vi "SetupDigitalPattern.vi"(6 "PatternfileName":string="Pattern.digipat", 8 "error in (no error)":errorcluster, 9 "DigitalWaveformName":string, 10 "pin list":string, 11 "IVI Refnum in":refnum<k15>) -> (0 "error out":errorcluster, 3 "IVI Refnum out":refnum<k15>)   [LabVIEW 2023]
uses:
  <instrlib>/niDigital/niDigital.llb/niDigital Load Specifications Levels and Timing (Single).vi
  <instrlib>/niDigital/niDigital.llb/niDigital Create Capture Waveform (Parallel).vi
  <instrlib>/niDigital/niDigital.llb/niDigital Create Source Waveform (Parallel).vi
  <instrlib>/niDigital/niDigital.llb/niDigital Write Source Waveform (Broadcast U32).vi
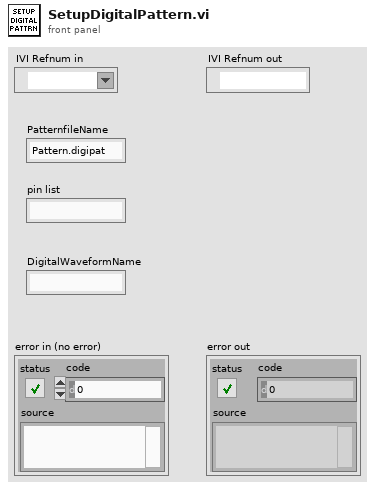
[diagram p1: front panel]
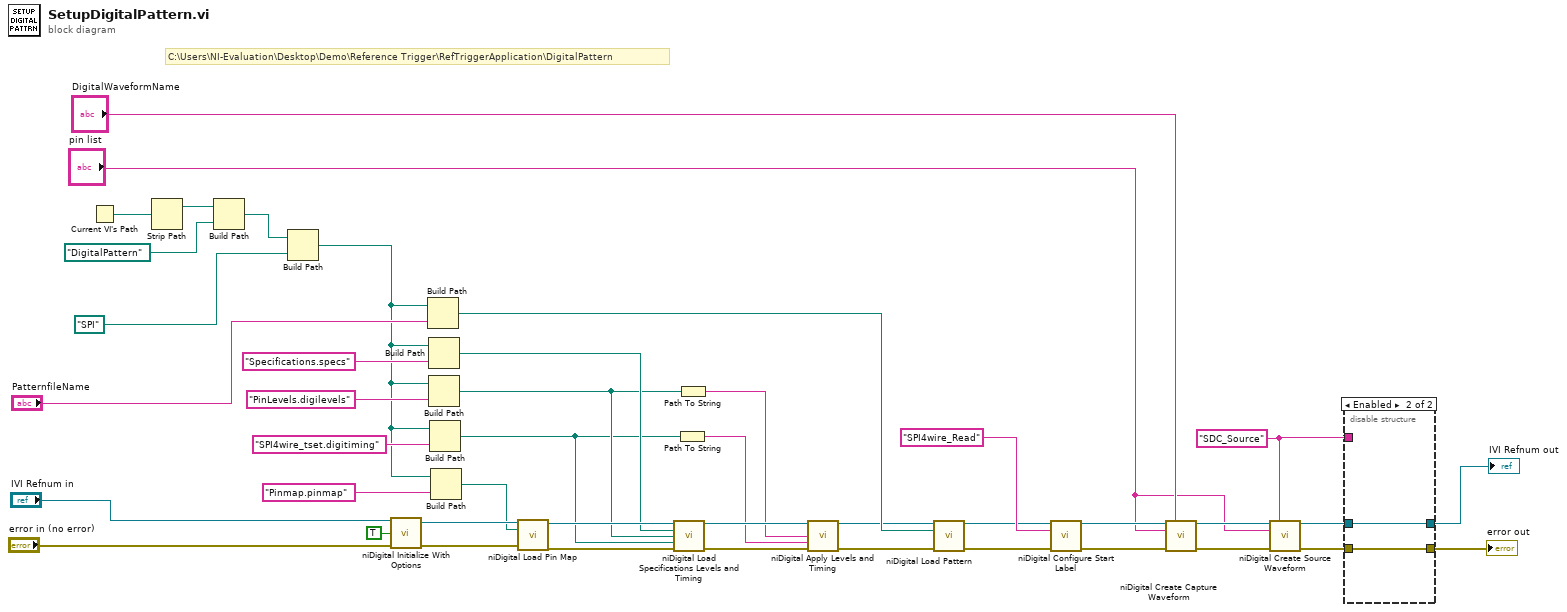
[diagram p0: block diagram]
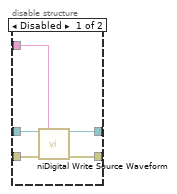
[diagram p2: hidden frame]
diagram:
  w5 = "SDC_Source" ("waveform name")
  # "C:\\Users\\NI-Evaluation\\Desktop\\Demo\\Reference Trigger\\RefTriggerApplication\\DigitalPattern"
  n1 = Current VI's Path() -> (path=w41:path)
  n2 = Strip Path(path=w41) -> (stripped path=w39:path)  [unwired: 1 out]
  n3 = Build Path(base path=w39, name or relative path=path "DigitalPattern") -> (appended path=w14:path)
  n4 = Build Path(base path=w14, name or relative path=path "SPI") -> (appended path=w15:path)
  n5 = call <instrlib>:"niDigital Initialize With Options.vi"("resource name"="IVI Refnum in", "reset (T)"=TRUE, "error in"="error in (no error)") -> ("instrument handle"=w36:refnum<k15>, "error out"=w35:errorcluster)  [unwired: 11 in]
  n6 = Build Path(base path=w15, name or relative path="PatternfileName") -> (appended path=w25:path)
  n7 = Build Path(base path=w15, name or relative path="Specifications.specs") -> (appended path=w28:path)
  n8 = Build Path(base path=w15, name or relative path="PinLevels.digilevels") -> (appended path=w12:path)
  n9 = Build Path(base path=w15, name or relative path="SPI4wire_tset.digitiming") -> (appended path=w10:path)
  n10 = Build Path(base path=w15, name or relative path="Pinmap.pinmap") -> (appended path=w27:path)
  n11 = call <instrlib>:"niDigital Load Pin Map.vi"("instrument handle"=w36, "pin map file"=w27, "error in"=w35) -> ("instrument handle out"=w38:refnum<k15>, "error out"=w37:errorcluster)  [unwired: 11 in]
  n12 = call-poly <instrlib>:"niDigital Load Specifications Levels and Timing.vi"("instrument handle"=w38, "specifications file path"=w28, "levels file path"=w12, "timing file path"=w10, "error in"=w37) -> ("instrument handle out"=w33:refnum<k15>, "error out"=w34:errorcluster)  [unwired: 9 in]
  n13 = Path To String(path=w10) -> (string=w9:string)
  n14 = Path To String(path=w12) -> (string=w11:string)
  n15 = call <instrlib>:"niDigital Apply Levels and Timing.vi"("instrument handle"=w33, "levels sheet"=w11, "timing sheet"=w9, "error in"=w34) -> ("instrument handle out"=w20:refnum<k15>, "error out"=w21:errorcluster)  [unwired: 10 in]
  n16 = call <instrlib>:"niDigital Load Pattern.vi"("instrument handle"=w20, "pattern file"=w25, "error in"=w21) -> ("instrument handle out"=w23:refnum<k15>, "error out"=w22:errorcluster)  [unwired: 11 in]
  n17 = call <instrlib>:"niDigital Configure Start Label.vi"("instrument handle"=w23, "start label"="SPI4wire_Read", "error in"=w22) -> ("instrument handle out"=w18:refnum<k15>, "error out"=w19:errorcluster)  [unwired: 11 in]
  n18 = call-poly <instrlib>:"niDigital Create Capture Waveform.vi"("instrument handle"=w18, "waveform name"="DigitalWaveformName", "pin list"="pin list", "error in"=w19) -> ("instrument handle out"=w8:refnum<k15>, "error out"=w7:errorcluster)  [unwired: 10 in]
  n19 = call-poly <instrlib>:"niDigital Create Source Waveform.vi"("instrument handle"=w8, "waveform name"=w5, "pin list"="pin list", "error in"=w7) -> ("instrument handle out"=w2:refnum<k15>, "error out"=w4:errorcluster)  [unwired: 10 in]
  n20 = disable-structure shown="Enabled" {
    disable-tunnel: w5 -> [w48 _]
    disable-tunnel: w4 -> [w47 w49]
    disable-tunnel: [w46 w49] -> w3
    disable-tunnel: w2 -> [w45 w50]
    disable-tunnel: [w44 w50] -> w1
    frame Disabled {
      n21 = call-poly <instrlib>:"niDigital Write Source Waveform.vi"("instrument handle"=w45, "waveform name"=w48, "error in"=w47) -> ("instrument handle out"=w44:refnum<k15>, "error out"=w46:errorcluster)  [unwired: 11 in]
    }
    frame Enabled {
    }
  }
  "IVI Refnum out" <- w1
  "error out" <- w3
